vi "JON_Query.vi"(0 "System no.":i32=1 min=1 max=4 step=1, 1 "JoystickID to query":i32[](array[numeric]), 3 "All joysticks?":bool, 5 "error in":errorcluster) -> (14 "Joystick status":i32[](array[numeric]), 19 "error out":errorcluster)   [LabVIEW 2020]
doc: "Returns activation status of queried joysticks connected to the controller.\n\nE-709: Only supported if E-709 is used inside C-867K012/K013."
panel:
  # "Returns activation status of queried joysticks connected to the controller."
  # "Query"
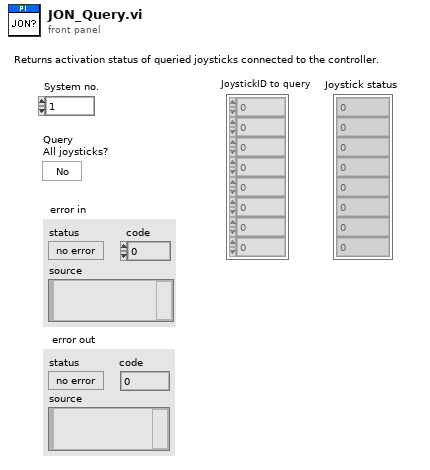
[diagram p1: front panel]
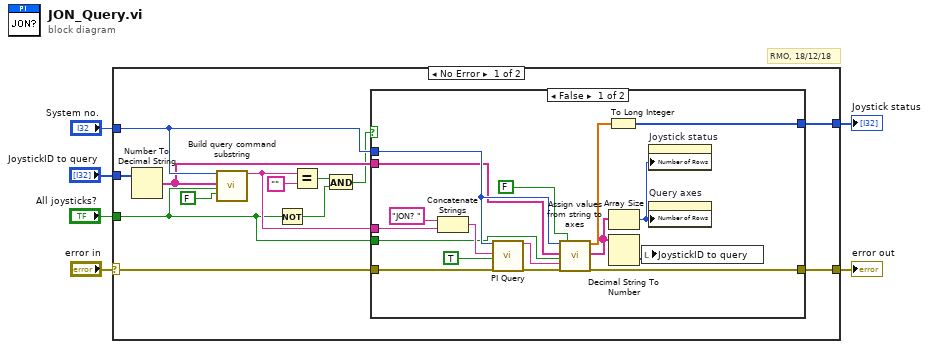
[diagram p0: block diagram]
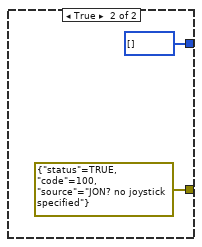
[diagram p2: hidden frame]
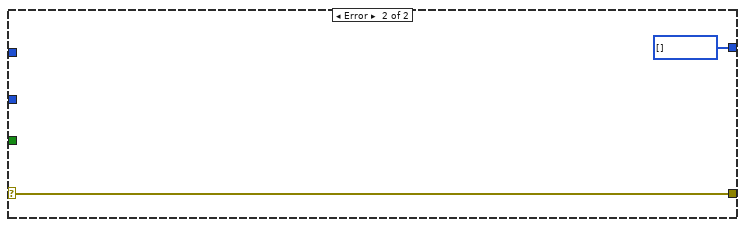
[diagram p3: hidden frame]
diagram:
  # "RMO, 18/12/18"
  n1 = case shown="No Error" "error in" {
    selector: "error in" -> [w9 w39]
    tunnel: [w12 i32[] [] ("Values")] -> w6
    tunnel: "JoystickID to query" -> [w11 _]
    tunnel: [w8 w39] -> w4
    tunnel: "System no." -> [w17 _]
    tunnel: "All joysticks?" -> [w16 _]
    frame No Error {
      n2 = Number To Decimal String(number=w11) -> (decimal integer string=w10:string[])  [unwired: 1 out]
      n3 = call "Build query command substring.vi"("System no."=w17, "Axes to query in"=w10, "Query\nAll axes?"=w16, "For all axes: use\nAxis identifier?"=FALSE ("For all axes: use\nAxis identifier?")) -> ("Command substring"=w18:string)  [unwired: 2 in, 13 out]
      n4 = Not(x=w16) -> (.not. x?=w14:bool)
      n5 = Equal?(x=w18, y="" ("x")) -> (x = y?=w15:bool)
      n6 = And(x=w15, y=w14) -> (x .and. y?=w7:bool)
      n7 = case shown="False" w7 {
        tunnel: w18 -> [w32 _]
        tunnel: w17 -> [w31 _]
        tunnel: w16 -> [w30 _]
        tunnel: [w29 i32[] []] -> w12
        tunnel: w10 -> [w26 _]
        tunnel: w9 -> [w23 _]
        tunnel: [w20 errorcluster {"status"=TRUE, "code"=100, "source"="JON? no joystick specified"} ("error out")] -> w8
        frame False {
          n8 = Concatenate Strings("JON? ", w32) -> (w34:string)
          n9 = call "PI Query.vi"("System no."=w31, "String to send"=w34, "Attach termination char.?"=TRUE ("Attach Linefeed?"), "error in"=w23) -> ("String read"=w21:string, "error out"=w22:errorcluster)  [unwired: 3 in, 11 out]
          n10 = call "Assign values from string to axes.vi"("System no."=w31, "Queried axes"=w26, "All axes queried?"=w30, "Input String"=w21, "error in"=w22, "Axes related?"=FALSE) -> ("Values"=w33:dbl[], "Queried axes out"=w25:string[], "error out"=w20:errorcluster)  [unwired: 3 in, 8 out]
          n11 = To Long Integer(number=w33) -> (32bit integer=w29:i32[])
          n12 = Array Size(array=w25) -> (size(s)=w28:i32)
          n13 = Decimal String To Number(string=w25) -> (number=w24:i32[])  [unwired: 3 out]
          n14 = local write "JoystickID to query"(w24) -> ()
          n15 = property on="Joystick status" class="Arr (strict)"("Number of Rows"=w28) -> ()  [unwired: 2 in, 2 out]
          n16 = property on="Query axes" class="Arr (strict)"("Number of Rows"=w28) -> ()  [unwired: 2 in, 2 out]
        }
        frame True {
        }
      }
    }
    frame Error {
    }
  }
  "error out" <- w4
  "Joystick status" <- w6
